vi "HP 4192 Impedance-1.vi"() -> ()   [LabVIEW 2010]
doc: "HP 4192A LF IMPEDANCE ANALYZER\n\nDEFAULTS: GPIB addr: 17\n Function A: Z/Y\n Function B: DEG\n Frequency: 100 Khz\n Circuit Mode: AUTO\n Trigger: INTERNAL\n Osc. Level: 1.0V\n DC Bias: OFF\n Bias Level: 0V\n\n\nGPIB PROGRAMMING NOTES: The command format consists of an ASCII string of control codes and numeric parameters. Commas act as seperators between individual commands. Whenever a numeric parameter is used, it is followed by 'EN,' signifying 'ENTER'. The 4192A is set to output an SRQ when a measurment is completed. The GPIB address is briefly shown in the 'DISPLAY A' window when the 4192A is first turned on. During remote operation, the 4192A front panel Remote LED will be activated verifying communication has been established. Consult the operation Manual Section 3, p68 for further description of the GPIB and control codes.\n\nINTERACTIVE OPERATION: The 4192A Virtural Instrument (VI) provides impedance measurments of circuits or components under test. 'FUNCTION A' selects the following measurments: Capacitance, Inductance, Resistance / Conductance, and Impedance / Addmittance. 'FUNCTION B' selects a characteristic of the measurment which includes: quality factor (Q), dissipation factor (D), resistance, or conductance. These parameters apply to L & C measurments. 'FUNCTION B' can also select Radians and Degrees which apply to Z/Y measurments. 'TEST SIGNAL FREQUENCY' has a range of 5Hz to 13Mhz. 'OSC LEVEL' has a range of 5mV to 1.1V. 'CIRCUIT MODE' selects between Auto mode, series circuits, and parallel circuits. The Series Mode applies to Z, R, and X measurments and the Parallel Mode applies to Y, G, and B measurments. The 'TRIGGER' control selects between Hold/Manual, External, and Internal Triggering. To operate the instrument interactively, select the desired options on the VI front panel and execute. The measurment results will be displayed in the 'DISPLAY A' and 'DISPLAY B' windows when execution is complete. Additionally, the 4192A can make bias or frequency sweep measurments using the '4192A Sweep' VI once the 4192A VI has been set up. The '4192A Sweep' provides bias and sweep options, start up and start down options, and selection between log or linear sweep.\n\nPROGRAMMATIC OPERATION: A example program is included in this package showing the 4192A and 4192A Sweep used programmatically. The following values can be used as inputs to the 4192A ICON; the ICON and connector pane are shown below:\n\n \n\n\nFREQUENCY: 5 to 13E6 Hz\n \nOSC. LEVEL: 5E-3 to 1.1V\n\nFUNCTION A INPUT: 0=Z/Y\n 1=R/G\n 2=L\n 3=C\n\nFUNCTION B INPUT: 0=DEG/Q\n 1=RAD/Q\n 2=R/G\n\nCIRCUIT MODE INPUT: 0=AUTO\n 1=SERIES\n 2=PARALLEL\n\nTRIGGER INPUT: 0=HOLD/MANUAL\n 1=EXTERNAL\n 2=INTERNAL\n\nBIAS: Binary Switch\n\nBIAS (V): -35 to 35V"
panel:
  in  "Scale of sweep freq":i16(slide) scale=0.0..1.0
  in  "Path and Filename of Data (Don't Forget .txt)\n\"C:\\filename\" saves on the C: drive":path
  out "XY Graph":cluster{"display B":dbl[], "display B":dbl[]}(graph)
  in  "function B (deg q:0)":i16(slide) scale=0.0..2.0 scale format="%.2f"
  in  "function A (z/y:0)":i16(slide)=1 scale=0.0..3.0
  out "capacitance\nvalue (F)":dbl format="%.3p"
  in  "step freq (Hz)":dbl=5000.0
  in  "stop freq (Hz)":dbl=1000000.0
  in  "start freq (Hz)":dbl=10000.0
  # "Z/Y"
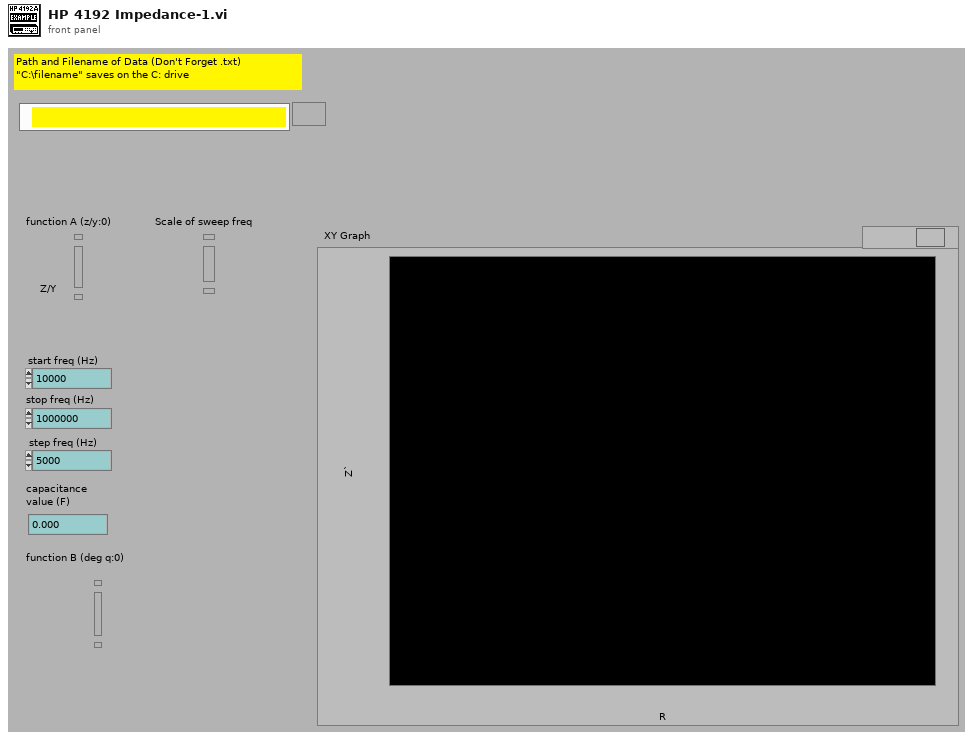
[diagram p1: front panel]
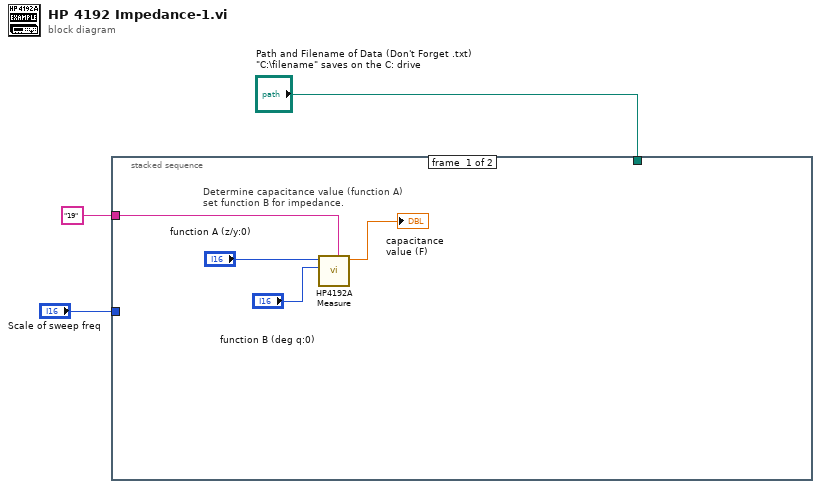
[diagram p0: block diagram]
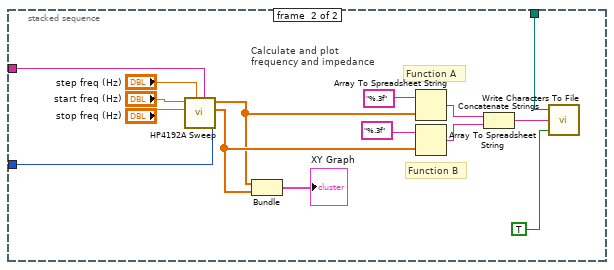
[diagram p2: hidden frame]
diagram:
  n1 = stacked-sequence {
    tunnel: "19" -> [w6 w21]
    tunnel: "Path and Filename of Data (Don't Forget .txt)\n\"C:\\filename\" saves on the C: drive" -> [_ w10]
    tunnel: "Scale of sweep freq" -> [_ w8]
    frame #0 {
      # "Determine capacitance value (function A)\nset function B for impedance."
      n2 = call "HP4192A Measure.vi"("GPIB addess"=w6, "function B (deg q:0)"="function B (deg q:0)", "function A (z/y:0)"="function A (z/y:0)") -> ("display A"=→"capacitance\nvalue (F)":dbl)  [unwired: 7 in, 1 out]
    }
    frame #1 {
      # "Function B"
      # "Function A"
      # "Calculate and plot\nfrequency and impedance"
      n3 = call "HP4192A Sweep.vi"("log sweep"=w8, "GPIB address"=w21, "step freq (Hz)"="step freq (Hz)", "stop freq (Hz)"="stop freq (Hz)", "start freq (Hz)"="start freq (Hz)") -> ("display B"=w14:dbl[], "display A"=w13:dbl[])  [unwired: 5 in]
      n4 = Bundle("display A"=w13, "display B"=w14) -> (→"XY Graph":cluster{"display A":dbl[], "display B":dbl[]})  [unwired: 1 in]
      n5 = Array To Spreadsheet String(array=w13, 3:"%.3f") -> (spreadsheet string=w16:string)  [unwired: 1 in]
      n6 = Array To Spreadsheet String(array=w14, 3:"%.3f") -> (spreadsheet string=w15:string)  [unwired: 1 in]
      n7 = Concatenate Strings(w16, w15) -> (w9:string)
      n8 = call <vilib>:"Write Characters To File.vi"("append to file? (new file:F)"=TRUE, "character string"=w9, "file path (dialog if empty)"=w10) -> ()  [unwired: 2 in, 1 out]
    }
  }
